vi "Rejestrator2_main.vi"() -> ()   [LabVIEW 2013]
uses:
  Kontrolki/GUI/AI_parametry.ctl
  Kontrolki/GUI/AI_wartosc.ctl
  Kontrolki/KartaDAQ/CONF AI HW config.ctl
  Kontrolki/GUI/DI_aktywacja.ctl
  Kontrolki/GUI/Encoder_parametry.ctl
  Kontrolki/GUI/Encoder_chanel.ctl
  Kontrolki/GUI/Rejestracja_szybka.ctl
  Kontrolki/GUI/Rejestracja_wolna.ctl
  Kontrolki/GUI/RejWol_konfig.ctl
  Kontrolki/GUI/RejWol_typ.ctl
  Kontrolki/GUI/Wolna_WykrNum.ctl
  Kontrolki/FVGs/FVG akcje podstawowa.ctl
  Kontrolki/KartaDAQ/CONF digital channel config.ctl
  Kontrolki/KartaDAQ/ACQ counter channel config.ctl
  Kontrolki/KartaDAQ/ACQ analog channel config.ctl
  Kontrolki/KartaDAQ/ACQ all read tasks.ctl
  Kontrolki/Przetwarzanie/Kanaly.ctl
  Kontrolki/FVGs/FVG GUI akcje.ctl
  <vilib>/DAQmx/configure/task.llb/DAQmx Start Task.vi
panel:
  out "Z karty DAQ":waveform(dbl)[](graph)
  out "przetworzone":waveform(dbl)[](graph)
  out "Skala":dbl=100.0 format="%#_13g"
  out "acq czas":dbl
  in  "Analog/Cyfr":bool
  out "Mnożniki wszystkie":dbl[](array[numeric])
  out "Mnożniki out":dbl[](array[numeric])
  in  "Tab Control":T1(tab)=enum."Konfiguracja"
  in  "Urządzenie":tag="Dev1"
  in  "AI HW conf array in":T2[](array[typedef])
  in  "Rejestracja wolna":T3={"WolnaStart"=FALSE, "WolnaPrzeglad"=FALSE, "Okres"=0.02, "Czas max"=120.0, "WolnaKonfiguracja"=FALSE, "Rej.1"={"Typ rejestracji"=enum."Wprost", "Kanały"=[1], "Opis"="Rej.X", "Aktywny"=FALSE, "Wolna Wykr num"=0}, "Rej.2"={"Typ rejestracji"=enum."Wprost", "Kanały"=[1], "Opis"="Rej.X", "Aktywny"=FALSE, "Wolna Wykr num"=0}, "Rej.3"={"Typ rejestracji"=enum."Wprost", "Kanały"=[1], "Opis"="Rej.X", "Aktywny"=FALSE, "Wolna Wykr num"=0}, "Rej.4"={"Typ rejestracji"=enum."Wprost", "Kanały"=[1], "Opis"="Rej.X", "Aktywny"=FALSE, "Wolna Wykr num"=0}, "Rej.5"={"Typ rejestracji"=enum."Wprost", "Kanały"=[1], "Opis"="Rej.X", "Aktywny"=FALSE, "Wolna Wykr num"=0}, "Rej.6"={"Typ rejestracji"=enum."Wprost", "Kanały"=[1], "Opis"="Rej.X", "Aktywny"=FALSE, "Wolna Wykr num"=0}, "Rej.7"={"Typ rejestracji"=enum."Wprost", "Kanały"=[1], "Opis"="Rej.X", "Aktywny"=FALSE, "Wolna Wykr num"=0}, "Rej.8"={"Typ rejestracji"=enum."Wprost", "Kanały"=[1], "Opis"="Rej.X", "Aktywny"=FALSE, "Wolna Wykr num"=0}} {"Rej.8"."Wolna Wykr num" items=["Brak", "Wykres 1", "Wykres 2", "Wykres 3", "Wykres 4"]; "Rej.7"."Wolna Wykr num" items=["Brak", "Wykres 1", "Wykres 2", "Wykres 3", "Wykres 4"]; "Rej.6"."Wolna Wykr num" items=["Brak", "Wykres 1", "Wykres 2", "Wykres 3", "Wykres 4"]; "Rej.5"."Wolna Wykr num" items=["Brak", "Wykres 1", "Wykres 2", "Wykres 3", "Wykres 4"]; "Rej.4"."Wolna Wykr num" items=["Brak", "Wykres 1", "Wykres 2", "Wykres 3", "Wykres 4"]; "Rej.3"."Wolna Wykr num" items=["Brak", "Wykres 1", "Wykres 2", "Wykres 3", "Wykres 4"]; "Rej.2"."Wolna Wykr num" items=["Brak", "Wykres 1", "Wykres 2", "Wykres 3", "Wykres 4"]; "Rej.1"."Wolna Wykr num" items=["Brak", "Wykres 1", "Wykres 2", "Wykres 3", "Wykres 4"]}
  in  "Rejestracja szybka":T7 {"Czas" scale=4.0..10.0}
  in  "Przemieszczenie":T8={"Wzorcowanie"=FALSE, "Zerowanie"=FALSE, "dT"=0.5, "d"=0.0, "v"=0.0, "a"=0.0, "Kanał"=enum."Kanał A"}
  in  "Kanały cyfrowe":T10={"DI1"=TRUE, "DI2"=TRUE, "DI3"=TRUE, "DI4"=TRUE, "DI1 Opis"="DI1", "DI2 Opis"="DI2", "DI3 Opis"="DI3", "DI4 Opis"="DI4", "DI1 Amplituda"=5.0, "DI2 Amplituda"=5.0, "DI3 Amplituda"=5.0, "DI4 Amplituda"=5.0}
  out "AI8":bool
  out "AI7":bool
  out "AI6":bool
  out "AI5":bool
  out "AI4":bool
  out "AI3":bool
  out "AI2":bool
  out "AI1":bool
  in  "Analog input":T11(tab) caption="Wejścia Analogowe (konfiguracja)"
  in  "AI_parametry 1":T12={"Numer"=1, "Opis"="Kanał 1", "Zakres"=enum."1000V", "Filtr"=FALSE, "Typ pomiaru"=enum."Wartość średnia", "Aktywny"=FALSE, "Wartość"={"X"="U", "[ ]"="V", "trans X"=1.0, "trans U"=1.0, "Z tabeli"=FALSE, "Opis"=""}} {"Numer" min=1 max=8 step=1}
  in  "AI_parametry 2":T12={"Numer"=1, "Opis"="Kanał 1", "Zakres"=enum."1000V", "Filtr"=FALSE, "Typ pomiaru"=enum."Wartość średnia", "Aktywny"=FALSE, "Wartość"={"X"="U", "[ ]"="V", "trans X"=1.0, "trans U"=1.0, "Z tabeli"=FALSE, "Opis"=""}} {"Numer" min=1 max=8 step=1}
  in  "AI_parametry 3":T12={"Numer"=1, "Opis"="Kanał 1", "Zakres"=enum."1000V", "Filtr"=FALSE, "Typ pomiaru"=enum."Wartość średnia", "Aktywny"=FALSE, "Wartość"={"X"="U", "[ ]"="V", "trans X"=1.0, "trans U"=1.0, "Z tabeli"=FALSE, "Opis"=""}} {"Numer" min=1 max=8 step=1}
  in  "AI_parametry 4":T12={"Numer"=1, "Opis"="Kanał 1", "Zakres"=enum."1000V", "Filtr"=FALSE, "Typ pomiaru"=enum."Wartość średnia", "Aktywny"=FALSE, "Wartość"={"X"="U", "[ ]"="V", "trans X"=1.0, "trans U"=1.0, "Z tabeli"=FALSE, "Opis"=""}} {"Numer" min=1 max=8 step=1}
  in  "AI_parametry 5":T12={"Numer"=1, "Opis"="Kanał 1", "Zakres"=enum."1000V", "Filtr"=FALSE, "Typ pomiaru"=enum."Wartość średnia", "Aktywny"=FALSE, "Wartość"={"X"="U", "[ ]"="V", "trans X"=1.0, "trans U"=1.0, "Z tabeli"=FALSE, "Opis"=""}} {"Numer" min=1 max=8 step=1}
  in  "AI_parametry 6":T12={"Numer"=1, "Opis"="Kanał 1", "Zakres"=enum."1000V", "Filtr"=FALSE, "Typ pomiaru"=enum."Wartość średnia", "Aktywny"=FALSE, "Wartość"={"X"="U", "[ ]"="V", "trans X"=1.0, "trans U"=1.0, "Z tabeli"=FALSE, "Opis"=""}} {"Numer" min=1 max=8 step=1}
  in  "AI_parametry 7":T12={"Numer"=1, "Opis"="Kanał 1", "Zakres"=enum."1000V", "Filtr"=FALSE, "Typ pomiaru"=enum."Wartość średnia", "Aktywny"=FALSE, "Wartość"={"X"="U", "[ ]"="V", "trans X"=1.0, "trans U"=1.0, "Z tabeli"=FALSE, "Opis"=""}} {"Numer" min=1 max=8 step=1}
  in  "AI_parametry 8":T12={"Numer"=1, "Opis"="Kanał 1", "Zakres"=enum."1000V", "Filtr"=FALSE, "Typ pomiaru"=enum."Wartość średnia", "Aktywny"=FALSE, "Wartość"={"X"="U", "[ ]"="V", "trans X"=1.0, "trans U"=1.0, "Z tabeli"=FALSE, "Opis"=""}} {"Numer" min=1 max=8 step=1}
  out "Enkoder Chart":waveform(dbl)[](graph)
  out "Szybka":waveform(dbl)[](graph)
  out "Array":dbl[](array[numeric])
  in  "StopBtn":bool
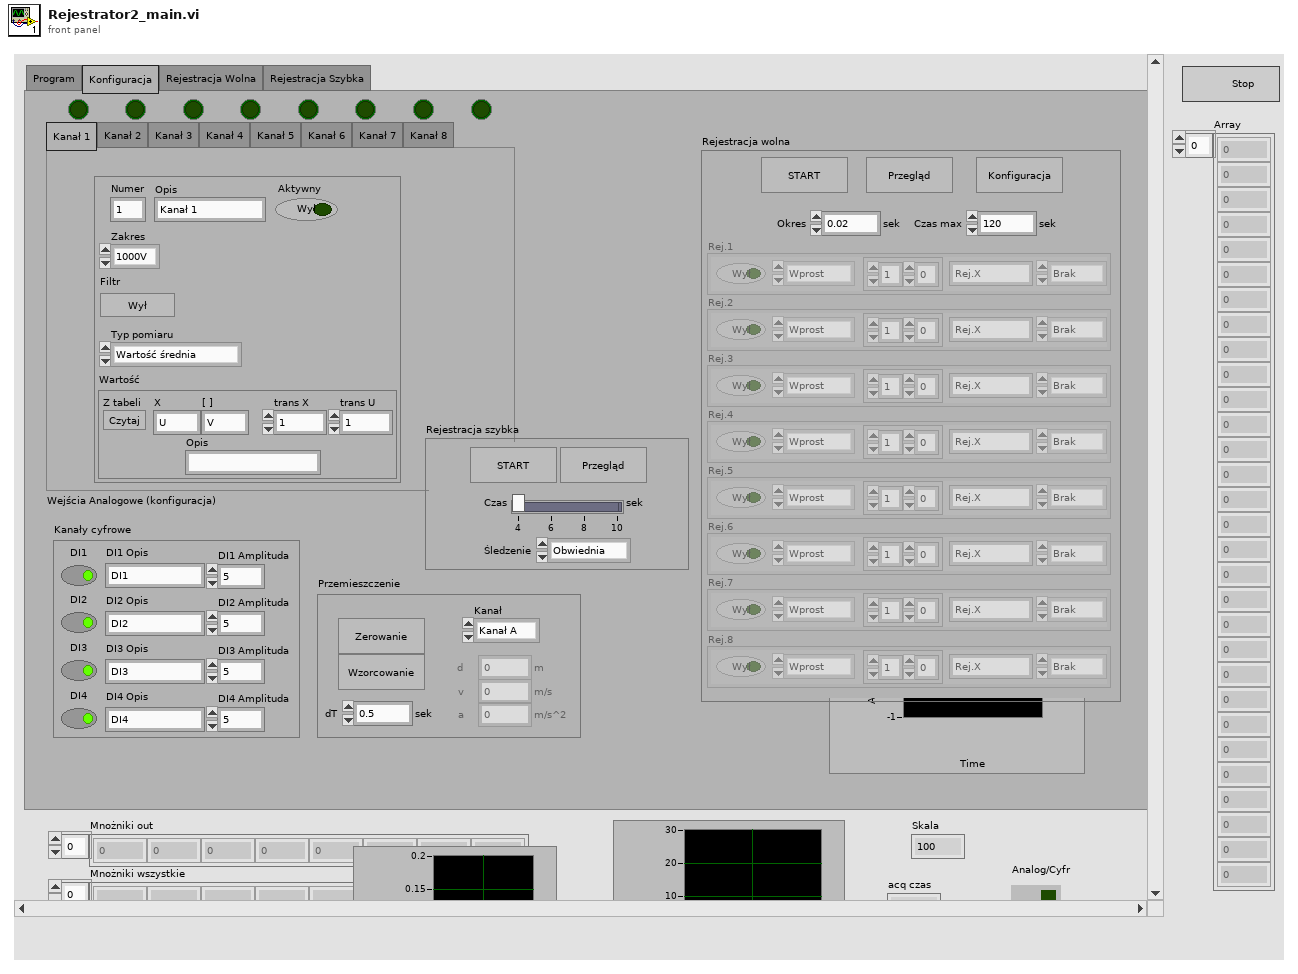
[diagram p1: front panel]
types:
  T1 = enum32{"Program", "Konfiguracja", "Rejestracja Wolna", "Rejestracja Szybka"}
  T2 = typedef "CONF AI HW config.ctl" = cluster{"Mux1":bool, "Mux2":bool, "Div1":bool, "Mux3":bool, "Div3":bool, "Div2":bool, "Filtr":bool, "reserved":bool}
  T3 = typedef "Rejestracja_wolna.ctl" = cluster{"WolnaStart":bool, "WolnaPrzeglad":bool, "Okres":dbl, "Czas max":dbl, "WolnaKonfiguracja":bool, "Rej.1":T4, "Rej.2":T4, "Rej.3":T4, "Rej.4":T4, "Rej.5":T4, "Rej.6":T4, "Rej.7":T4, "Rej.8":T4}
  T4 = typedef "RejWol_konfig.ctl" = cluster{"Typ rejestracji":T5, "Kanały":i32[], "Opis":string, "Aktywny":bool, "Wolna Wykr num":T6}
  T5 = typedef "RejWol_typ.ctl" = enum16{"Wprost", "Moduł", "Kwadrat", "Iloczyn", "Faza"}
  T6 = typedef "Wolna_WykrNum.ctl" = u16
  T7 = typedef "Rejestracja_szybka.ctl" = cluster{"SzybkaStart":bool, "SzybkaPrzeglad":bool, "Śledzenie":enum16{"Obwiednia", "Migawka"}, "Czas":i32}
  T8 = typedef "Encoder_parametry.ctl" = cluster{"Wzorcowanie":bool, "Zerowanie":bool, "dT":dbl, "d":dbl, "v":dbl, "a":dbl, "Kanał":T9}
  T9 = typedef "Encoder_chanel.ctl" = enum16{"Kanał A", "Kanał B"}
  T10 = typedef "DI_aktywacja.ctl" = cluster{"DI1":bool, "DI2":bool, "DI3":bool, "DI4":bool, "DI1 Opis":string, "DI2 Opis":string, "DI3 Opis":string, "DI4 Opis":string, "DI1 Amplituda":dbl, "DI2 Amplituda":dbl, "DI3 Amplituda":dbl, "DI4 Amplituda":dbl}
  T11 = enum32{"Kanał 1", "Kanał 2", "Kanał 3", "Kanał 4", "Kanał 5", "Kanał 6", "Kanał 7", "Kanał 8"}
  T12 = typedef "AI_parametry.ctl" = cluster{"Numer":u8, "Opis":string, "Zakres":enum16{"1000V", "300V", "30V", "3V", "0,3V"}, "Filtr":bool, "Typ pomiaru":enum16{"Wartość średnia", "Średnia wyprostowana", "Wartość skuteczna"}, "Aktywny":bool, "Wartość":T13}
  T13 = typedef "AI_wartosc.ctl" = cluster{"X":string, "[ ]":string, "trans X":dbl, "trans U":dbl, "Z tabeli":bool, "Opis":string}
  T14 = typedef "Kanaly.ctl" = cluster{"Analogowe":waveform(dbl)[], "Cyfrowe":waveform(dbl)[], "Zwarcie":waveform(dbl)[], "Enkoder":waveform(dbl)[]}
  T15 = typedef "ACQ all read tasks.ctl" = cluster{"Enkoder X ref":refnum<k21>, "Enkoder Y ref":refnum<k21>, "Generator ref":refnum<k21>, "Analog ref":refnum<k21>}
  T16 = typedef "ACQ analog channel config.ctl" = cluster{"Analog IN":string, "Digital IN":string, "Cont IN":string}
  T17 = typedef "ACQ counter channel config.ctl" = cluster{"Enkoder X":string, "Enkoder Y":string, "Generator":string, "Generator OUT":string}
  T18 = typedef "CONF digital channel config.ctl" = cluster{"SEnable":string, "SData":string, "SClock":string}
  T19 = typedef "FVG akcje podstawowa.ctl" = enum16{"GET", "SET"}
  T20 = typedef "FVG GUI akcje.ctl" = enum16{"GET", "SET AI Aktywny", "SET DI Aktywny"}
  T21 = typedef "CONF Digital Refnum.ctl" = cluster{"Sen Ref out":refnum<k21>, "Data Ref out":refnum<k21>}
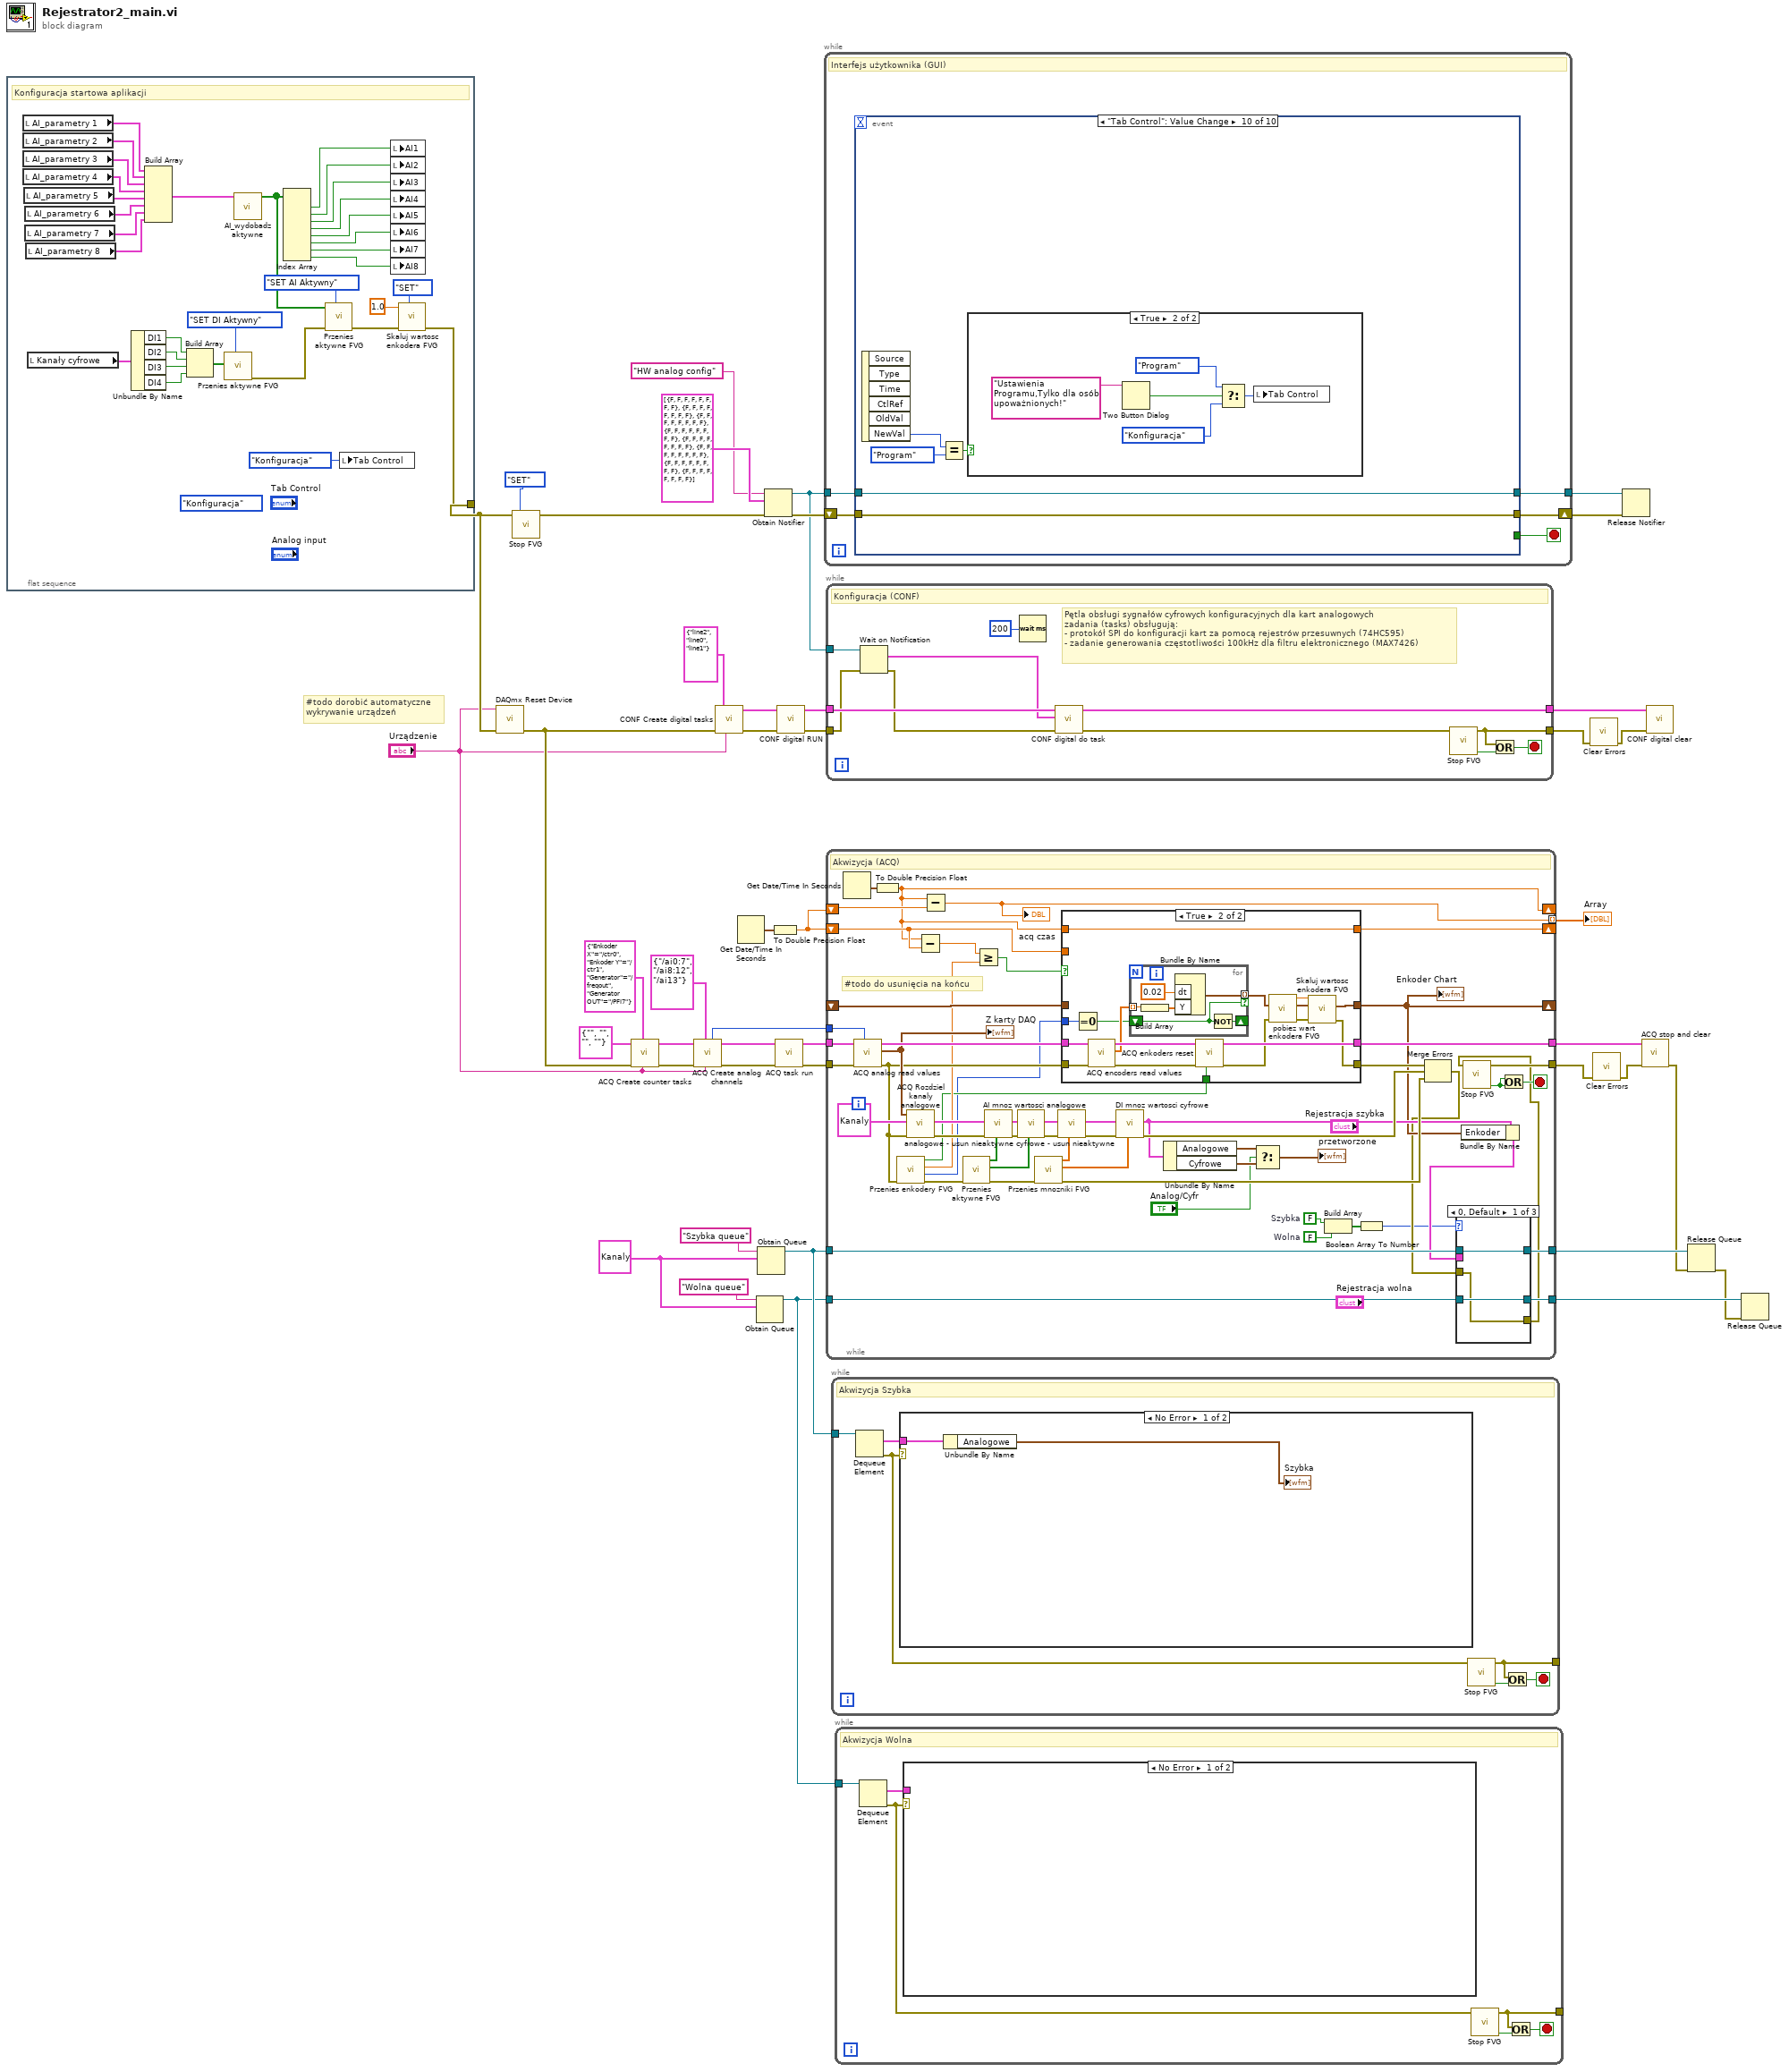
[diagram p0: block diagram]
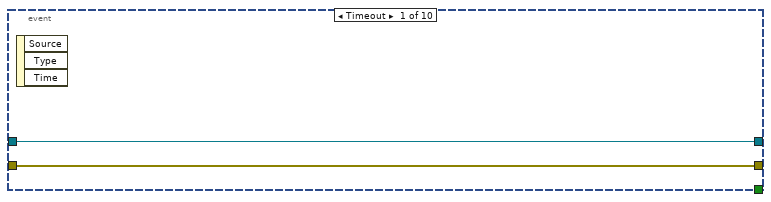
[diagram p4: hidden frame]
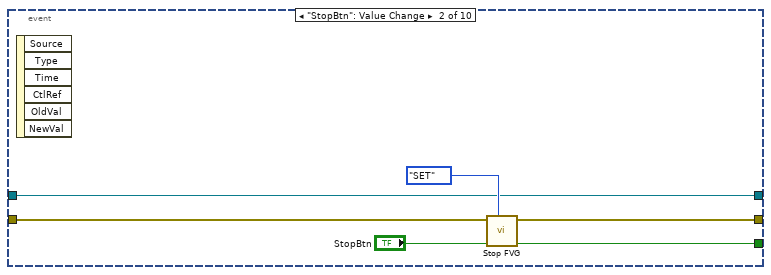
[diagram p5: hidden frame]
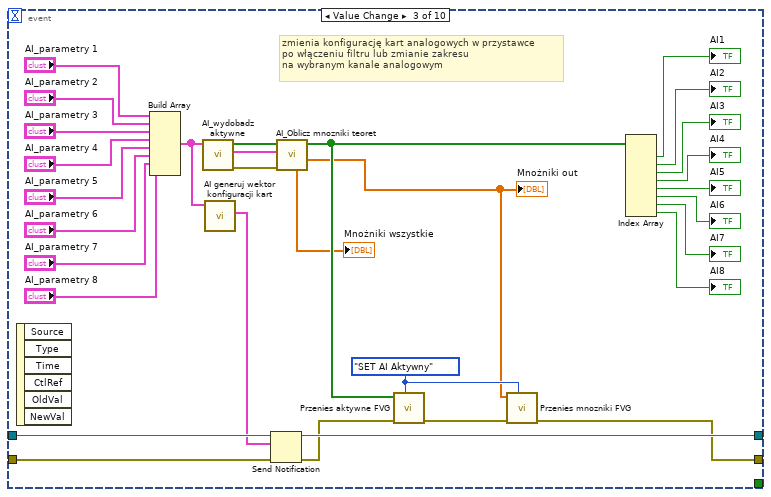
[diagram p6: hidden frame]
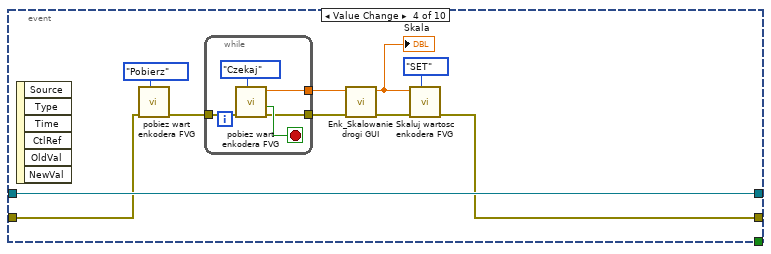
[diagram p7: hidden frame]
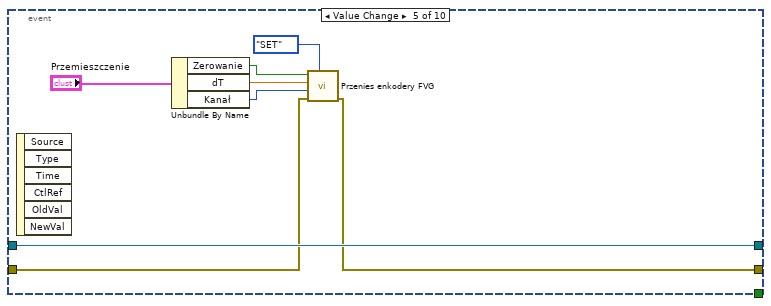
[diagram p8: hidden frame]
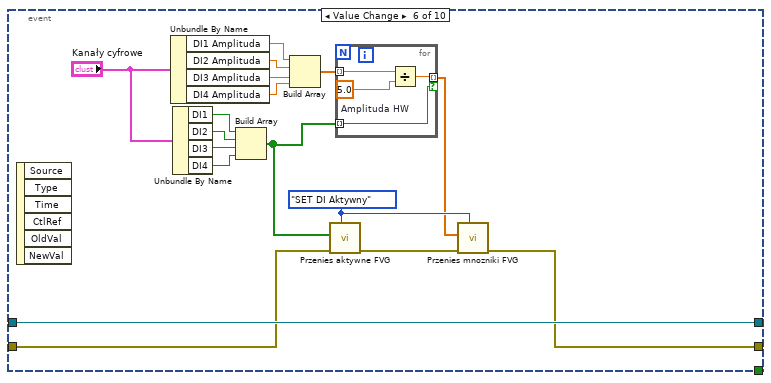
[diagram p9: hidden frame]
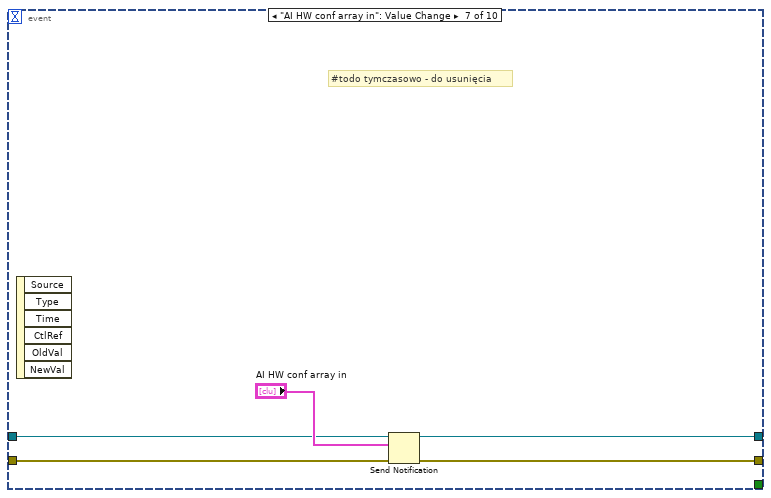
[diagram p10: hidden frame]
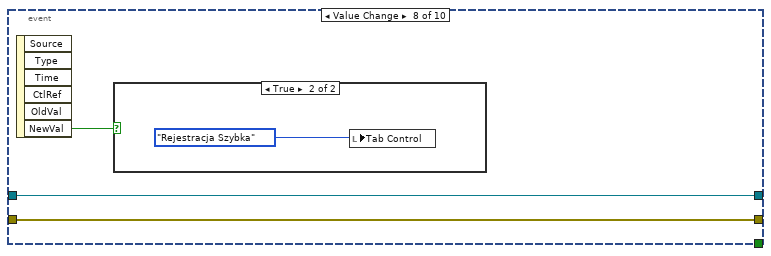
[diagram p11: hidden frame]
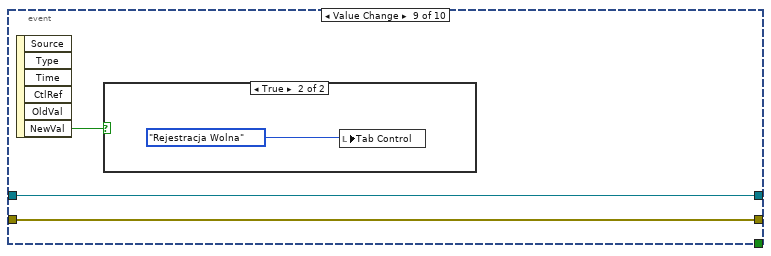
[diagram p13: hidden frame]
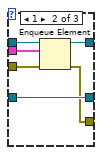
[diagram p16: hidden frame]
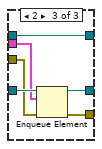
[diagram p17: hidden frame]
diagram:
  w7 = T14 data[32432B] ("Kanaly")
  # "#todo dorobić automatyczne\nwykrywanie urządzeń"
  n1 = flat-sequence {
    tunnel: [w47] -> w26
    frame #0 {
      (unwired) T1."Konfiguracja" ("Tab Control")
      # "Konfiguracja startowa aplikacji"
      n2 = local read "AI_parametry 1"() -> (w75:T12)
      n3 = local read "AI_parametry 2"() -> (w74:T12)
      n4 = local read "AI_parametry 3"() -> (w73:T12)
      n5 = local read "AI_parametry 4"() -> (w72:T12)
      n6 = local read "AI_parametry 5"() -> (w71:T12)
      n7 = local read "AI_parametry 6"() -> (w70:T12)
      n8 = local read "AI_parametry 7"() -> (w69:T12)
      n9 = local read "AI_parametry 8"() -> (w68:T12)
      n10 = local read "Kanały cyfrowe"() -> (w51:T10)
      n11 = Unbundle By Name(w51) -> ("DI1"=w57:bool, "DI2"=w56:bool, "DI3"=w55:bool, "DI4"=w54:bool)
      n12 = Build Array(w75, w74, w73, w72, w71, w70, w69, w68) -> (w50:T12[])
      n13 = Build Array(w57, w56, w55, w54) -> (w53:bool[])
      n14 = call "Przenies aktywne FVG.vi"("Akcja (Get)"=FVG_GUI_akcje."SET DI Aktywny", "DI Aktywne in"=w53) -> ("error out"=w52:errorcluster)  [unwired: 7 in, 2 out]
      n15 = call "AI_wydobadz aktywne.vi"("AI param array in"=w50) -> ("Aktywne Array out"=w49:bool[])  [unwired: 8 in, 2 out]
      n16 = Index Array(array=w49) -> (element #1=w67:bool, element #2=w66:bool, element #3=w65:bool, element #4=w64:bool, element #5=w63:bool, element #6=w62:bool, element #7=w61:bool, element #8=w60:bool)  [unwired: 8 in]
      n17 = call "Przenies aktywne FVG.vi"("Akcja (Get)"=FVG_GUI_akcje."SET AI Aktywny", "error in (no error)"=w52, "AI Aktywne in"=w49) -> ("error out"=w48:errorcluster)  [unwired: 6 in, 2 out]
      n18 = local write "Tab Control"(T1."Konfiguracja" ("Tab Control")) -> ()
      n19 = local write "AI1"(w67) -> ()
      n20 = local write "AI2"(w66) -> ()
      n21 = local write "AI3"(w65) -> ()
      n22 = local write "AI4"(w64) -> ()
      n23 = local write "AI5"(w63) -> ()
      n24 = local write "AI6"(w62) -> ()
      n25 = local write "AI7"(w61) -> ()
      n26 = local write "AI8"(w60) -> ()
      n27 = call "Skaluj wartosc enkodera FVG.vi"("Akcja (GET)"=FVG_akcje_podstawowa."SET", "error in (no error)"=w48, "Skala"=1.0) -> ("error out"=w47:errorcluster)  [unwired: 7 in, 1 out]
    }
  }
  n28 = call <vilib>:"DAQmx Reset Device.vi"("device in"="Urządzenie", "error in"=w26) -> ("error out"=w12:errorcluster)  [unwired: 13 in]
  n29 = call "Stop FVG.vi"("Akcja (GET)"=FVG_akcje_podstawowa."SET", "error in (no error)"=w26) -> ("error out"=w37:errorcluster)  [unwired: 8 in, 1 out]
  n30 = call "ACQ Create counter tasks.vi"("device in"="Urządzenie", "Config Counter channels"=T17 {"Enkoder X"="/ctr0", "Enkoder Y"="/ctr1", "Generator"="/freqout", "Generator OUT"="/PFI7"}, "error in (no error)"=w12, "All Read tasks in"=T15 {"Enkoder X ref"="", "Enkoder Y ref"="", "Generator ref"="", "Analog ref"=""}) -> ("error out"=w28:errorcluster, "All Read tasks out"=w27:T15)  [unwired: 5 in, 1 out]
  n31 = call "ACQ Create analog channels.vi"("device in"="Urządzenie", "Config analog chanells"=T16 {"Analog IN"="/ai0:7", "Digital IN"="/ai8:12", "Cont IN"="/ai13"}, "error in (no error)"=w28, "All Read tasks in"=w27) -> ("error out"=w13:errorcluster, "All Read tasks out"=w25:T15, "samples per channel"=w22:i32)  [unwired: 4 in, 1 out]
  n32 = call "CONF Create digital tasks.vi"("device in"="Urządzenie", "Config Digital Channels"=T18 {"SEnable"="line2", "SData"="line0", "SClock"="line1"}, "error in (no error)"=w12) -> ("error out"=w42:errorcluster, "Digital ref out"=w41:T21)  [unwired: 7 in]
  n33 = Get Date/Time In Seconds() -> (seconds since 1Jan1904=w15:timestamp)
  n34 = Obtain Queue(name (unnamed)="Wolna queue", element data type=w7) -> (queue out=w1:refnum<queue>)  [unwired: 3 in, 2 out]
  n35 = Obtain Queue(name (unnamed)="Szybka queue", element data type=w7) -> (queue out=w2:refnum<queue>)  [unwired: 3 in, 2 out]
  n36 = Obtain Notifier(name (unnamed)="HW analog config", notification data type=T2[] [{"Mux1"=FALSE, "Mux2"=FALSE, "Div1"=FALSE, "Mux3"=FALSE, "Div3"=FALSE, "Div2"=FALSE, "Filtr"=FALSE, "reserved"=FALSE}, {"Mux1"=FALSE, "Mux2"=FALSE, "Div1"=FALSE, "Mux3"=FALSE, "Div3"=FALSE, "Div2"=FALSE, "Filtr"=FALSE, "reserved"=FALSE}, {"Mux1"=FALSE, "Mux2"=FALSE, "Div1"=FALSE, "Mux3"=FALSE, "Div3"=FALSE, "Div2"=FALSE, "Filtr"=FALSE, "reserved"=FALSE}, {"Mux1"=FALSE, "Mux2"=FALSE, "Div1"=FALSE, "Mux3"=FALSE, "Div3"=FALSE, "Div2"=FALSE, "Filtr"=FALSE, "reserved"=FALSE}, {"Mux1"=FALSE, "Mux2"=FALSE, "Div1"=FALSE, "Mux3"=FALSE, "Div3"=FALSE, "Div2"=FALSE, "Filtr"=FALSE, "reserved"=FALSE}, {"Mux1"=FALSE, "Mux2"=FALSE, "Div1"=FALSE, "Mux3"=FALSE, "Div3"=FALSE, "Div2"=FALSE, "Filtr"=FALSE, "reserved"=FALSE}, {"Mux1"=FALSE, "Mux2"=FALSE, "Div1"=FALSE, "Mux3"=FALSE, "Div3"=FALSE, "Div2"=FALSE, "Filtr"=FALSE, "reserved"=FALSE}, {"Mux1"=FALSE, "Mux2"=FALSE, "Div1"=FALSE, "Mux3"=FALSE, "Div3"=FALSE, "Div2"=FALSE, "Filtr"=FALSE, "reserved"=FALSE}] ("AI HW conf array in"), error in (no error)=w37) -> (notifier out=w32:refnum<notifier>, error out=w38:errorcluster)  [unwired: 1 in, 1 out]
  n37 = To Double Precision Float(number=w15) -> (double precision float=w14:dbl)
  n38 = call "ACQ task run.vi"("error in (no error)"=w13, "All Read tasks in"=w25) -> ("error out"=w24:errorcluster, "All Read tasks out"=w23:T15)  [unwired: 7 in, 1 out]
  n39 = call "CONF digital RUN.vi"("error in (no error)"=w42, "Digital ref in"=w41) -> ("error out"=w43:errorcluster, "Digital ref out"=w40:T21)  [unwired: 8 in]
  n40 = while {
    shift-right: [w80] -> w34
    shift-left: w38 -> [w79]
    tunnel: w32 -> [w78]
    tunnel: [w77] -> w33
    stop <- w81 stop-if-true
    # "Interfejs użytkownika (GUI)"
    n41 = event shown="[9] \"Tab Control\": Value Change" {
      selector: _ -> [_ _ _ _ _ _ _ _ _ _]
      dyn-events: _ -> [_ _ _ _ _ _ _ _ _ _]
      timeout: _ -> [_ _ _ _ _ _ _ _ _ _]
      tunnel: [_ w86 _ _ _ _ _ _ _ _] -> w81
      tunnel: [w83 w88 w92 w123 w140 w152 w168 w172 w176 w182] -> w80
      tunnel: w79 -> [w83 w87 w118 w124 w141 w159 w169 w172 w176 w182]
      tunnel: w78 -> [w82 w84 w120 w130 w143 w160 w166 w171 w175 w181]
      tunnel: [w82 w84 w119 w130 w143 w160 w165 w171 w175 w181] -> w77
      event Timeout {
        n42 = event-data() -> ()  [unwired: 1 in, 3 out]
      }
      event "StopBtn": Value Change {
        n43 = event-data() -> ()  [unwired: 1 in, 6 out]
        n44 = call "Stop FVG.vi"("Akcja (GET)"=FVG_akcje_podstawowa."SET", "Stop in (F)"="StopBtn", "error in (no error)"=w87) -> ("Stop out"=w86:bool, "error out"=w88:errorcluster)  [unwired: 7 in]
      }
      event Value Change {
        w91 = FVG_GUI_akcje."SET AI Aktywny" ("Akcja")
        # "zmienia konfigurację kart analogowych w przystawce\npo włączeniu filtru lub zmianie zakresu\nna wybranym kanale analogowym"
        n45 = event-data() -> ()  [unwired: 1 in, 6 out]
        n46 = Build Array("AI_parametry 1", "AI_parametry 2", "AI_parametry 3", "AI_parametry 4", "AI_parametry 5", "AI_parametry 6", "AI_parametry 7", "AI_parametry 8") -> (w99:T12[])
        n47 = call "AI_wydobadz aktywne.vi"("AI param array in"=w99) -> ("error out"=w95:errorcluster, "AI param aktywne out"=w96:T12[], "Aktywne Array out"=w98:bool[])  [unwired: 8 in]
        n48 = call "AI generuj wektor konfiguracji kart.vi"("AI_param in"=w99) -> ("HW konfig"=w117:T2[])  [unwired: 9 in, 1 out]
        n49 = Send Notification(notification=w117, notifier=w120, error in (no error)=w118) -> (notifier out=w119:refnum<notifier>, error out=w108:errorcluster)
        n50 = call "AI_Oblicz mnozniki teoret.vi"("error in (no error)"=w95, "AI param aktywne in"=w96, "Aktywne Array in"=w98) -> ("Mnożniki out"=w90:dbl[], "Aktywne Array out"=w97:bool[], "Mnożniki wszystkie out"=→"Mnożniki wszystkie":dbl[])  [unwired: 5 in, 1 out]
        "Mnożniki out" <- w90
        n51 = call "Przenies aktywne FVG.vi"("Akcja (Get)"=w91, "error in (no error)"=w108, "AI Aktywne in"=w97) -> ("error out"=w93:errorcluster)  [unwired: 6 in, 2 out]
        n52 = call "Przenies mnozniki FVG.vi"("Akcja (Get)"=w91, "error in (no error)"=w93, "AI Mnozniki in"=w90) -> ("error out"=w92:errorcluster)  [unwired: 6 in, 2 out]
        n53 = Index Array(array=w97) -> (element #1=→"AI1":bool, element #2=→"AI2":bool, element #3=→"AI3":bool, element #4=→"AI4":bool, element #5=→"AI5":bool, element #6=→"AI6":bool, element #7=→"AI7":bool, element #8=→"AI8":bool)  [unwired: 8 in]
      }
      event Value Change {
        n54 = event-data() -> ()  [unwired: 1 in, 6 out]
        n55 = call "pobiez wart enkodera FVG.vi"("Akcja (Pobrano)"=enum16{"Pobierz", "Pobrano", "Czekaj"}."Pobierz", "error in (no error)"=w124) -> ("error out"=w128:errorcluster)  [unwired: 6 in, 3 out]
        n56 = while {
          tunnel: w128 -> [w133]
          tunnel: [w132] -> w127
          tunnel: [w131] -> w122
          stop <- w134 stop-if-true
          n57 = call "pobiez wart enkodera FVG.vi"("Akcja (Pobrano)"=enum16{"Pobierz", "Pobrano", "Czekaj"}."Czekaj", "error in (no error)"=w133) -> ("error out"=w132:errorcluster, "Flaga"=w134:bool, "Impulsy Out"=w131:dbl)  [unwired: 6 in, 1 out]
        }
        n58 = call "Enk_Skalowanie drogi GUI.vi"("error in (no error)"=w127, "Droga In"=w122) -> ("error out"=w126:errorcluster, "Skala"=w121:dbl)  [unwired: 8 in]
        "Skala" <- w121
        n59 = call "Skaluj wartosc enkodera FVG.vi"("Akcja (GET)"=FVG_akcje_podstawowa."SET", "error in (no error)"=w126, "Skala"=w121) -> ("error out"=w123:errorcluster)  [unwired: 7 in, 1 out]
      }
      event Value Change {
        n60 = event-data() -> ()  [unwired: 1 in, 6 out]
        n61 = Unbundle By Name("Przemieszczenie") -> ("Zerowanie"=w139:bool, "dT"=w138:dbl, "Kanał"=w137:T9)
        n62 = call "Przenies enkodery FVG.vi"("Akcja (Get)"=FVG_akcje_podstawowa."SET", "error in (no error)"=w141, "Kanał in"=w137, "dT in"=w138, "Zerowanie in"=w139) -> ("error out"=w140:errorcluster)  [unwired: 3 in, 3 out]
      }
      event Value Change {
        w154 = FVG_GUI_akcje."SET DI Aktywny" ("Akcja (Get)")
        n63 = event-data() -> ()  [unwired: 1 in, 6 out]
        n64 = Unbundle By Name("Kanały cyfrowe") -> ("DI1 Amplituda"=w150:dbl, "DI2 Amplituda"=w149:dbl, "DI3 Amplituda"=w148:dbl, "DI4 Amplituda"=w147:dbl)
        n65 = Unbundle By Name("Kanały cyfrowe") -> ("DI1"=w158:bool, "DI2"=w157:bool, "DI3"=w156:bool, "DI4"=w155:bool)
        n66 = Build Array(w158, w157, w156, w155) -> (w145:bool[])
        n67 = Build Array(w150, w149, w148, w147) -> (w146:dbl[])
        n68 = call "Przenies aktywne FVG.vi"("Akcja (Get)"=w154, "error in (no error)"=w159, "DI Aktywne in"=w145) -> ("error out"=w153:errorcluster)  [unwired: 6 in, 2 out]
        n69 = for {
          tunnel: w146 -> [w164] mode=indexing
          tunnel: w145 -> [w162] mode=indexing
          tunnel: [w163] -> w144 mode=indexing if=w162
          w161 = 5.0  # Amplituda HW
          n70 = Divide(x=w164, y=w161) -> (x/y=w163:dbl)
        }
        n71 = call "Przenies mnozniki FVG.vi"("Akcja (Get)"=w154, "error in (no error)"=w153, "DI Mnozniki in"=w144) -> ("error out"=w152:errorcluster)  [unwired: 6 in, 2 out]
      }
      event "AI HW conf array in": Value Change {
        # "#todo tymczasowo - do usunięcia"
        n72 = event-data() -> ()  [unwired: 1 in, 6 out]
        n73 = Send Notification(notification="AI HW conf array in", notifier=w166, error in (no error)=w169) -> (notifier out=w165:refnum<notifier>, error out=w168:errorcluster)
      }
      event Value Change {
        n74 = event-data() -> ("NewVal"=w170:bool)  [unwired: 1 in, 5 out]
        n75 = case shown="True" w170 {
          frame False {
          }
          frame True {
            n76 = local write "Tab Control"(T1."Rejestracja Szybka" ("Tab Control")) -> ()
          }
        }
      }
      event Value Change {
        n77 = event-data() -> ("NewVal"=w174:bool)  [unwired: 1 in, 5 out]
        n78 = case shown="True" w174 {
          frame False {
          }
          frame True {
            n79 = local write "Tab Control"(T1."Rejestracja Wolna" ("Tab Control")) -> ()
          }
        }
      }
      event "Tab Control": Value Change {
        n80 = event-data() -> ("NewVal"=w179:T1)  [unwired: 1 in, 5 out]
        n81 = Equal?(x=w179, y=T1."Program" ("Tab Control")) -> (x = y?=w178:bool)
        n82 = case shown="True" w178 {
          frame False {
          }
          frame True {
            n83 = Two Button Dialog(message="Ustawienia Programu,Tylko dla osób upoważnionych!") -> (T button?=w186:bool)  [unwired: 2 in]
            n84 = Select(t=T1."Program" ("Tab Control"), s=w186, f=T1."Konfiguracja" ("Tab Control")) -> (s? t:f=w183:T1)
            n85 = local write "Tab Control"(w183) -> ()
          }
        }
      }
    }
  }
  n86 = while {
    tunnel: w24 -> [w242]
    tunnel: w23 -> [w241]
    tunnel: w22 -> [w244]
    tunnel: [w225] -> w20
    tunnel: [w239] -> w21
    shift-right: [w234] -> _
    shift-left: w14 -> [w233]
    shift-right: [w231] -> _
    shift-left: w14 -> [w232]
    tunnel: [w230] -> w11 mode=indexing
    shift-right: [w199] -> _
    shift-left: _ -> [w207]
    tunnel: w2 -> [w198]
    tunnel: w1 -> [w197]
    tunnel: [w195] -> w6
    tunnel: [w194] -> w5
    stop <- w243 stop-if-true
    w190 = FALSE  # Wolna
    w191 = FALSE  # Szybka
    # "#todo do usunięcia na końcu"
    # "Akwizycja (ACQ)"
    n87 = Get Date/Time In Seconds() -> (seconds since 1Jan1904=w237:timestamp)
    n88 = call "ACQ analog read values.vi"("samples per channel"=w244, "error in (no error)"=w242, "Tasks ref in"=w241) -> ("error out"=w204:errorcluster, "data"=w229:waveform(dbl)[], "Tasks ref out"=w240:T15)  [unwired: 6 in]
    "Z karty DAQ" <- w229
    n89 = To Double Precision Float(number=w237) -> (double precision float=w231:dbl)
    n90 = call "Przenies enkodery FVG.vi"("error in (no error)"=w204) -> ("error out"=w205:errorcluster, "Kanał out"=w201:T9, "dT out"=w203:dbl, "Zerowanie out"=w202:bool)  [unwired: 7 in]
    n91 = call "ACQ Rozdziel kanaly analogowe.vi"("error in (no error)"=w204, "Kanaly in"=T14 data[32432B] ("Kanaly"), "data"=w229) -> ("error out"=w222:errorcluster, "Kanaly out"=w227:T14)  [unwired: 7 in]
    n92 = Subtract(x=w231, y=w233) -> (x-y=w236:dbl)
    n93 = Subtract(x=w231, y=w232) -> (x-y=w230:dbl)
    "acq czas" <- w230
    n94 = call "Przenies aktywne FVG.vi"("error in (no error)"=w205) -> ("error out"=w220:errorcluster, "DI Aktywne out"=w223:bool[], "AI Aktywne out"=w224:bool[])  [unwired: 8 in]
    n95 = Greater Or Equal?(x=w236, y=w203) -> (x >= y?=w235:bool)
    n96 = call "analogowe - usun nieaktywne.vi"("Kanaly aktywne"=w224, "error in (no error)"=w222, "Kanaly in"=w227) -> ("error out"=w221:errorcluster, "Kanaly out"=w226:T14)  [unwired: 7 in]
    n97 = call "cyfrowe - usun nieaktywne.vi"("Kanaly aktywne"=w223, "error in (no error)"=w221, "Kanaly in"=w226) -> ("error out"=w218:errorcluster, "Kanaly out"=w216:T14)  [unwired: 7 in]
    n98 = call "Przenies mnozniki FVG.vi"("error in (no error)"=w220) -> ("error out"=w219:errorcluster, "DI Mnozniki out"=w212:dbl[], "AI Mnozniki out"=w217:dbl[])  [unwired: 8 in]
    n99 = call "AI mnoz wartosci analogowe.vi"("Mnozniki in"=w217, "error in (no error)"=w218, "Kanaly in"=w216) -> ("error out"=w215:errorcluster, "Kanaly out"=w214:T14)  [unwired: 6 in, 1 out]
    n100 = case shown="True" w235 {
      tunnel: w204 -> [w262 w280]
      tunnel: w240 -> [w263 w279]
      tunnel: [w262 w267] -> w200
      tunnel: [w263 w277] -> w239
      tunnel: w233 -> [w261 _]
      tunnel: [w261 w278] -> w234
      tunnel: w231 -> [_ w278]
      tunnel: w202 -> [_ w274]
      tunnel: w207 -> [w260 _]
      tunnel: w201 -> [_ w272]
      tunnel: [w260 w266] -> w199
      frame False {
      }
      frame True {
        n101 = Equal To 0?(x=w272) -> (x = 0?=w271:bool)
        n102 = call "ACQ encoders read values.vi"("error in (no error)"=w280, "Tasks ref in"=w279) -> ("error out"=w276:errorcluster, "Encoders out"=w273:dbl[], "Tasks ref out"=w275:T15)  [unwired: 7 in]
        n103 = for {
          tunnel: w273 -> [w286] mode=indexing
          tunnel: [w283] -> w269 mode=indexing if=w281
          shift-right: [w282] -> _
          shift-left: w271 -> [w281]
          n104 = Build Array(w286) -> (w285:dbl[])
          n105 = Bundle By Name("dt"=0.02, "Y"=w285) -> (w283:waveform(dbl))  [unwired: 1 in]
          n106 = Not(x=w281) -> (.not. x?=w282:bool)
        }
        n107 = call "ACQ enkoders reset.vi"("Reset"=w274, "error in (no error)"=w276, "Tasks ref in"=w275) -> ("error out"=w268:errorcluster, "Tasks ref out"=w277:T15)  [unwired: 7 in]
        n108 = call "pobiez wart enkodera FVG.vi"("error in (no error)"=w268, "Impulsy In"=w269) -> ("error out"=w270:errorcluster, "Impulsy Out wfm"=w265:waveform(dbl)[], "Impulsy Out"=w264:dbl)  [unwired: 6 in, 1 out]
        n109 = call "Skaluj wartosc enkodera FVG.vi"("error in (no error)"=w270, "Impulsy In"=w265, "Skala"=w264) -> ("error out"=w267:errorcluster, "Impulsy Out"=w266:waveform(dbl)[])  [unwired: 7 in]
      }
    }
    "Enkoder Chart" <- w199
    n110 = call "DI mnoz wartosci cyfrowe.vi"("Mnozniki in"=w212, "error in (no error)"=w215, "Kanaly in"=w214) -> ("error out"=w213:errorcluster, "Kanaly out"=w206:T14)  [unwired: 6 in, 1 out]
    n111 = Unbundle By Name(w206) -> ("Analogowe"=w211:waveform(dbl)[], "Cyfrowe"=w210:waveform(dbl)[])
    n112 = Select(t=w211, s="Analog/Cyfr", f=w210) -> (s? t:f=→"przetworzone":waveform(dbl)[])
    n113 = Build Array(w191, w190) -> (w189:bool[])
    n114 = Boolean Array To Number(Boolean array=w189) -> (number=w188:u32)
    n115 = Merge Errors(w200, w213, w219) -> (w193:errorcluster)
    n116 = Bundle By Name(cluster=w206, "Enkoder"=w199) -> (w196:T14)
    n117 = case shown="0, Default" w188 {
      tunnel: w198 -> [w247 w253 w254]
      tunnel: w197 -> [w246 w249 w259]
      tunnel: w196 -> [_ w252 w255]
      tunnel: [w247 w251 w254] -> w195
      tunnel: [w246 w249 w258] -> w194
      tunnel: w193 -> [w245 w250 w256]
      tunnel: [w245 w248 w257] -> w192
      frame 0, Default {
      }
      frame 1 {
        n118 = Enqueue Element(queue=w253, element=w252, error in (no error)=w250) -> (queue out=w251:refnum<queue>, error out=w248:errorcluster)  [unwired: 1 in, 1 out]
      }
      frame 2 {
        n119 = Enqueue Element(queue=w259, element=w255, error in (no error)=w256) -> (queue out=w258:refnum<queue>, error out=w257:errorcluster)  [unwired: 1 in, 1 out]
      }
    }
    n120 = call "Stop FVG.vi"("error in (no error)"=w192) -> ("Stop out"=w238:bool, "error out"=w225:errorcluster)  [unwired: 9 in]
    n121 = Or(x=w238, y=w238) -> (x .or. y?=w243:bool)
  }
  "Array" <- w11
  n122 = while {
    tunnel: w43 -> [w292]
    tunnel: w40 -> [w296]
    tunnel: [w289] -> w31
    tunnel: [w295] -> w39
    tunnel: w32 -> [w293]
    stop <- w288 stop-if-true
    # "Pętla obsługi sygnałów cyfrowych konfiguracyjnych dla kart analogowych\nzadania (tasks) obsługują:\n- protokół SPI do konfiguracji kart za pomocą rejestrów przesuwnych (74HC595)\n- zadanie generowania częstotliwości 100kHz dla filtru elektronicznego (MAX7426)"
    # "Konfiguracja (CONF)"
    n123 = Wait on Notification(notifier=w293, error in (no error)=w292) -> (notification=w287:T2[], error out=w291:errorcluster)  [unwired: 2 in, 2 out]
    n124 = Wait (ms)(milliseconds to wait=u32 200) -> ()  [unwired: 1 out]
    n125 = call "CONF digital do task.vi"("error in (no error)"=w291, "AI HW conf array in"=w287, "Digital ref in"=w296) -> ("error out"=w294:errorcluster, "Digital ref out"=w295:T21)  [unwired: 6 in, 1 out]
    n126 = call "Stop FVG.vi"("error in (no error)"=w294) -> ("Stop out"=w290:bool, "error out"=w289:errorcluster)  [unwired: 9 in]
    n127 = Or(x=w289, y=w290) -> (x .or. y?=w288:bool)
  }
  n128 = while {
    tunnel: w2 -> [w303]
    tunnel: [w300] -> _
    stop <- w299 stop-if-true
    # "Akwizycja Szybka"
    n129 = Dequeue Element(queue=w303) -> (element=w298:T14, error out=w302:errorcluster)  [unwired: 2 in, 2 out]
    n130 = case shown="No Error" w302 {
      tunnel: w298 -> [w305 _]
      frame No Error {
        n131 = Unbundle By Name(w305) -> ("Analogowe"=→"Szybka":waveform(dbl)[])
      }
      frame Error {
      }
    }
    n132 = call "Stop FVG.vi"("error in (no error)"=w302) -> ("Stop out"=w301:bool, "error out"=w300:errorcluster)  [unwired: 9 in]
    n133 = Or(x=w300, y=w301) -> (x .or. y?=w299:bool)
  }
  n134 = while {
    tunnel: w1 -> [w311]
    tunnel: [w308] -> _
    stop <- w307 stop-if-true
    # "Akwizycja Wolna"
    n135 = Dequeue Element(queue=w311) -> (element=w306:T14, error out=w310:errorcluster)  [unwired: 2 in, 2 out]
    n136 = case shown="No Error" w310 {
      tunnel: w306 -> [_ _]
      frame No Error {
      }
      frame Error {
      }
    }
    n137 = call "Stop FVG.vi"("error in (no error)"=w310) -> ("Stop out"=w309:bool, "error out"=w308:errorcluster)  [unwired: 9 in]
    n138 = Or(x=w308, y=w309) -> (x .or. y?=w307:bool)
  }
  n139 = call <vilib>:"Clear Errors.vi"("error in (no error)"=w31) -> ("error out"=w30:errorcluster)  [unwired: 6 in]
  n140 = call <vilib>:"Clear Errors.vi"("error in (no error)"=w20) -> ("error out"=w19:errorcluster)  [unwired: 6 in]
  n141 = Release Notifier(notifier=w33, error in (no error)=w34) -> ()  [unwired: 1 in, 3 out]
  n142 = call "ACQ stop and clear.vi"("error in (no error)"=w19, "Tasks ref in"=w21) -> ("error out"=w4:errorcluster)  [unwired: 9 in]
  n143 = call "CONF digital clear.vi"("error in (no error)"=w30, "Digital ref out"=w39) -> ()  [unwired: 9 in, 1 out]
  n144 = Release Queue(queue=w6, error in (no error)=w4) -> (error out=w3:errorcluster)  [unwired: 1 in, 2 out]
  n145 = Release Queue(queue=w5, error in (no error)=w3) -> ()  [unwired: 1 in, 3 out]
